vi "IOScan_StringConsts.vi"() -> ()   [LabVIEW 2016]
panel:
  in  "DNL_Major":string="Major"
  in  "DNL_Unconfigured":string="Unconfigured"
  in  "DNL_Minor":string="Minor"
  in  "DNL_Ignore":string="Ignore"
  in  "DNL_Custom":string="Custom"
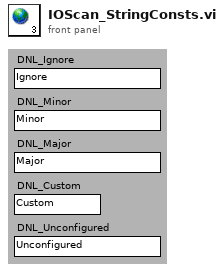
[diagram p1: front panel]
diagram:
